vi "Tiling.vi"() -> ()   [LabVIEW 2020]
uses:
  <vilib>/DAQmx/write.llb/DAQmx Write (Analog 1D Wfm NChan NSamp).vi
  <vilib>/DAQmx/create/channels.llb/DAQmx Create Channel (AO-Voltage-Basic).vi
  <vilib>/DAQmx/configure/timing.llb/DAQmx Timing (Use Waveform).vi
  <vilib>/DAQmx/miscellaneous.llb/DAQmx Fill In Error Info.vi
  <vilib>/measure/NI_MABase.lvlib
panel:
  in  "Z step size (um) 4":dbl=0.2
  in  "Sawtooth Offset 4":dbl=0.005 format="%.2p"
  in  "Camera trigger delay (degrees) 4":dbl=-5.0 format="%.2p"
  out "# Samples written per channel 4":u32=1000
  in  "Stop Analog Signal 4":bool
  in  "Sawtooth Phase 4":dbl=180.0 format="%.2p"
  in  "Sawtooth Amplitude 4":dbl=0.24 format="%.2p"
  in  "Z step size (um) 3":dbl=0.2
  in  "Sawtooth Offset 3":dbl=0.005 format="%.2p"
  in  "Camera trigger delay (degrees) 3":dbl=-5.0 format="%.2p"
  out "# Samples written per channel 3":u32=1000
  in  "Stop Analog Signal 3":bool
  in  "Sawtooth Phase 3":dbl=180.0 format="%.2p"
  in  "Sawtooth Amplitude 3":dbl=0.24 format="%.2p"
  in  "Z step size (um) 2":dbl=0.2
  in  "Sawtooth Offset 2":dbl=0.005 format="%.2p"
  in  "Camera trigger delay (degrees) 2":dbl=-5.0 format="%.2p"
  out "# Samples written per channel 2":u32=1000
  in  "Stop Analog Signal 2":bool
  in  "Sawtooth Phase 2":dbl=180.0 format="%.2p"
  in  "Sawtooth Amplitude 2":dbl=0.24 format="%.2p"
  out "Z Position":dbl
  out "X Position":dbl=3.2928906249999996
  out "Y Position":dbl=0.7058199999999999
  out "Error out":errorcluster
  in  "Disable All Axis":bool
  in  "Sawtooth Amplitude":dbl=0.24 format="%.2p"
  in  "Sawtooth Phase":dbl=180.0 format="%.2p"
  in  "Stop Analog Signal":bool
  out "# Samples written per channel":u32=1000
  in  "Exposure time (ms)":dbl=1000.0
  in  "Camera trigger delay (degrees)":dbl=-5.0 format="%.2p"
  in  "Sawtooth Offset":dbl=0.005 format="%.2p"
  in  "Z step size (um)":dbl=0.2
  out "Number of Slices":dbl=100.0
  in  "Input will be multiplied by 5":dbl=20.0
  out "GetFirmwareVersion 2":string="3.03\r"
  out "Connected":bool=TRUE
  in  "SPIIPLUSCOM660Lib.IAsyncChannel":refnum<k7>
  # "2x2 Tiling, 1.3mm x 1.3 mm x 0.5 mm Voxel"
  # "Zstack parameters"
  # "Parameters for analog input to Voice coil"
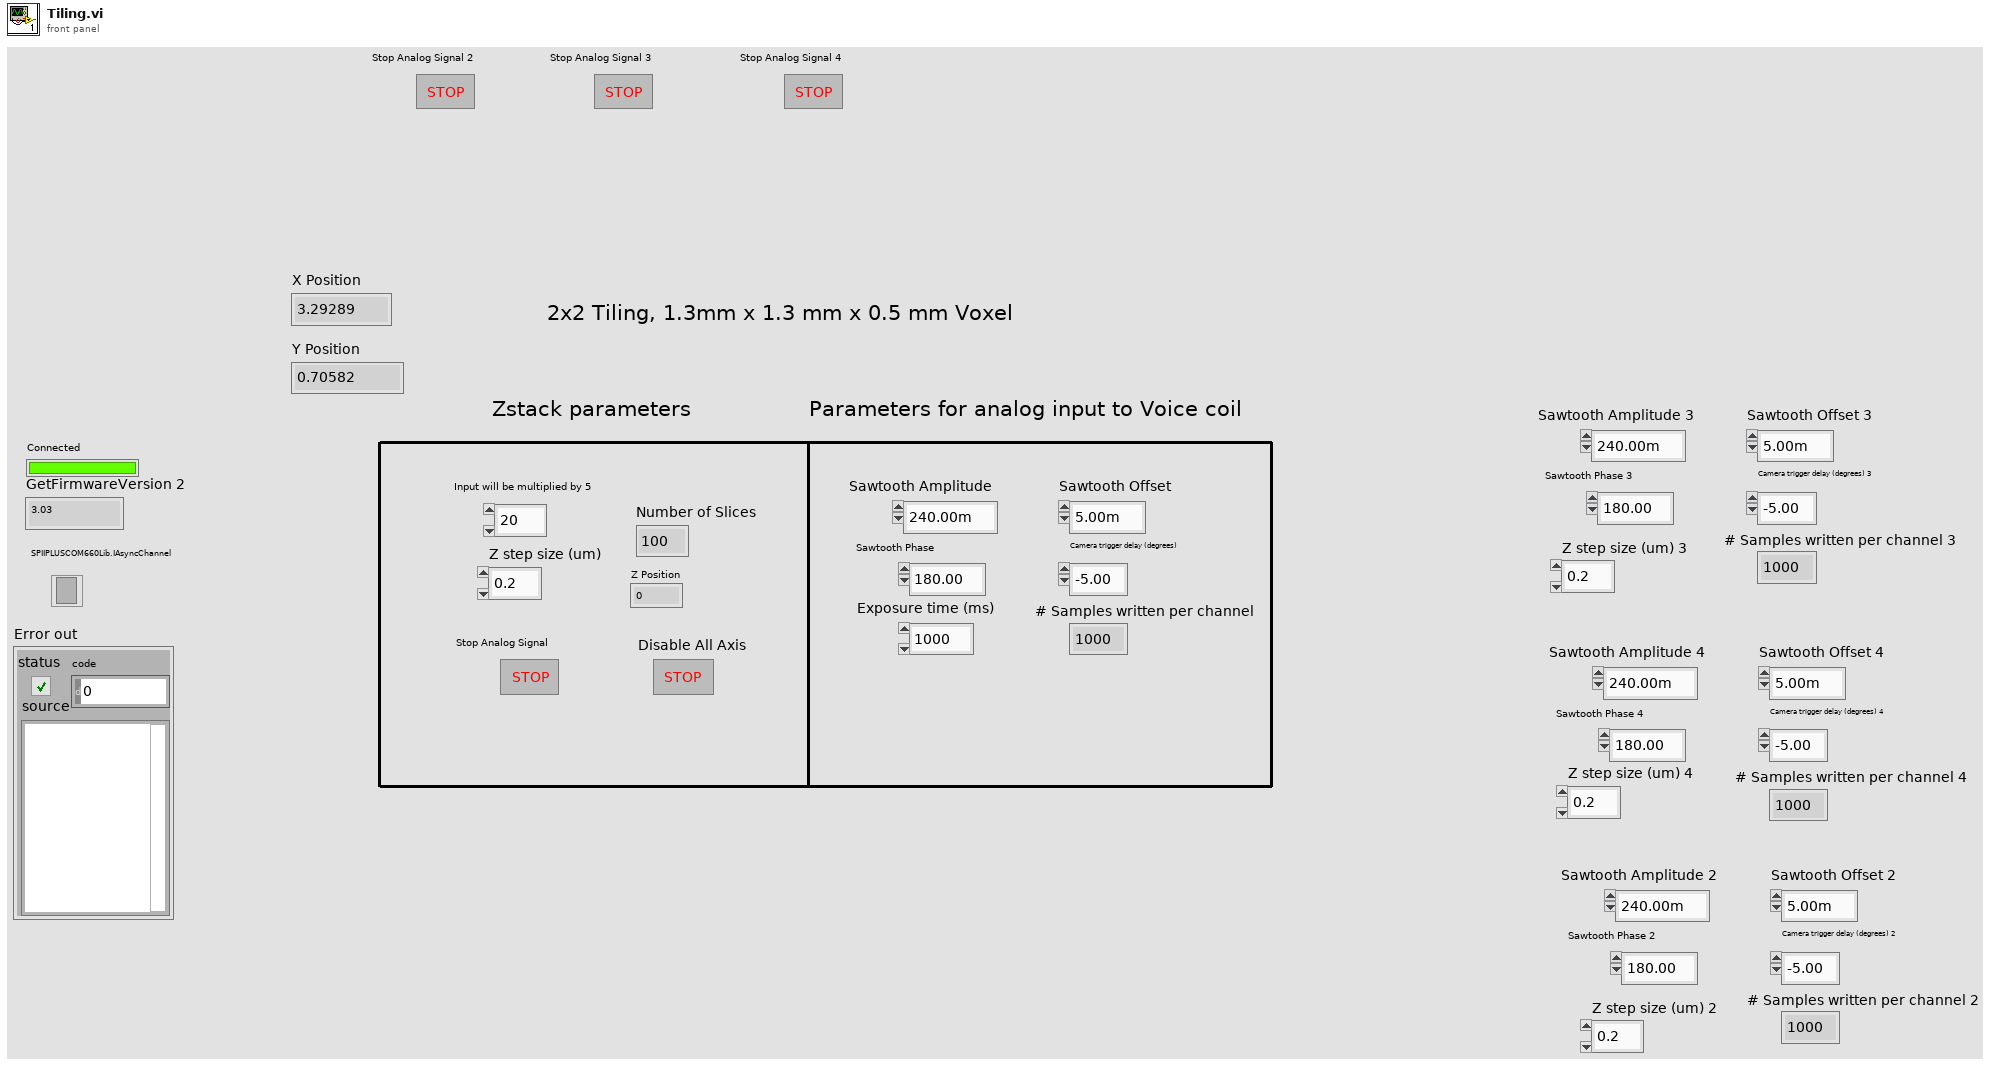
[diagram p1: front panel]
diagram:
  n1 = flat-sequence {
    tunnel: [w12] -> w9
    tunnel: [w11] -> w8
    tunnel: w9 -> [w22]
    tunnel: w8 -> [w21]
    tunnel: [w19] -> w7
    tunnel: [w18] -> w6
    tunnel: w7 -> [w29]
    tunnel: w6 -> [w30]
    tunnel: [w39] -> w5
    tunnel: [w38] -> w4
    tunnel: [w37] -> w3
    tunnel: w5 -> [w570]
    tunnel: w4 -> [w569]
    tunnel: [w568] -> w2
    tunnel: [w567] -> w1
    tunnel: w3 -> [_]
    tunnel: w2 -> [w572]
    tunnel: w1 -> [w571]
    frame #0 {
      n2 = Automation Open(Automation Refnum="SPIIPLUSCOM660Lib.IAsyncChannel") -> (Automation Refnum=w17:refnum<k7>)  [unwired: 3 in, 1 out]
      n3 = property class="IAsyncChannel"(reference=w17) -> (reference out=w16:refnum<k7>, error out=w10:errorcluster, "ACSC_SOCKET_STREAM_PORT"=w14:i32)  [unwired: 1 in]
      n4 = invoke class="IAsyncChannel" method="OpenCommEthernetTCP"(reference=w16, error in=w10, "Address"="10.0.0.100", "Port"=w14) -> (reference out=w12:refnum<k7>, error out=w11:errorcluster)  [unwired: 1 in, 3 out]
    }
    frame #1 {
      n5 = invoke class="IAsyncChannel" method="GetFirmwareVersion"(reference=w22, error in=w21, "CallType"=u64 0, "pWait"=variant) -> (reference out=w19:refnum<k7>, error out=w18:errorcluster, "GetFirmwareVersion"=w24:string)  [unwired: 1 in, 2 out]
      "GetFirmwareVersion 2" <- w24
      n6 = Empty String/Path?(string/path=w24) -> (empty?=w23:bool)
      n7 = Not(x=w23) -> (.not. x?=→"Connected":bool)
    }
    frame #2 {
      n8 = property class="IAsyncChannel"(reference=w29, error in=w30) -> (reference out=w36:refnum<k7>, error out=w35:errorcluster, "ACSC_AXIS_2"=w37:i32)
      n9 = property class="IAsyncChannel"(reference=w29, error in=w30) -> (reference out=w34:refnum<k7>, error out=w33:errorcluster, "ACSC_AXIS_0"=w32:i32)
      n10 = property class="IAsyncChannel"(reference=w29, error in=w30) -> (reference out=w28:refnum<k7>, error out=w27:errorcluster, "ACSC_AXIS_1"=w31:i32)
      n11 = while {
        shift-right: [w177] -> w39
        shift-left: w36 -> [w158]
        shift-right: [w176] -> w38
        shift-left: w35 -> [w157]
        tunnel: w37 -> [w151]
        tunnel: w32 -> [w44]
        tunnel: w31 -> [w51]
        shift-right: [w74] -> _
        shift-left: w33 -> [w163]
        shift-right: [w75] -> _
        shift-left: w34 -> [w164]
        shift-right: [w77] -> _
        shift-left: w28 -> [w79]
        shift-right: [w76] -> _
        shift-left: w27 -> [w78]
        stop <- "Disable All Axis" stop-if-true
        n12 = invoke class="IAsyncChannel" method="GetRPosition"(reference=w79, error in=w78, "Axis"=w51, "CallType"=u64 0, "pWait"=variant) -> (reference out=w57:refnum<k7>, error out=w56:errorcluster, "GetRPosition"=→"Y Position":dbl)  [unwired: 1 in, 3 out]
        n13 = invoke class="IAsyncChannel" method="GetRPosition"(reference=w164, error in=w163, "Axis"=w44, "CallType"=u64 0, "pWait"=variant) -> (reference out=w61:refnum<k7>, error out=w60:errorcluster, "GetRPosition"=→"X Position":dbl)  [unwired: 1 in, 3 out]
        n14 = invoke class="IAsyncChannel" method="GetRPosition"(reference=w158, error in=w157, "Axis"=w151, "CallType"=u64 0, "pWait"=variant) -> (reference out=w156:refnum<k7>, error out=w155:errorcluster, "GetRPosition"=→"Z Position":dbl)  [unwired: 1 in, 3 out]
        n15 = invoke class="IAsyncChannel" method="Enable"(reference=w57, error in=w56, "Axis"=w51, "CallType"=u64 0, "pWait"=variant) -> (reference out=w55:refnum<k7>, error out=w54:errorcluster)  [unwired: 1 in, 4 out]
        n16 = invoke class="IAsyncChannel" method="Enable"(reference=w61, error in=w60, "Axis"=w44, "CallType"=u64 0, "pWait"=variant) -> (reference out=w48:refnum<k7>, error out=w47:errorcluster)  [unwired: 1 in, 4 out]
        n17 = invoke class="IAsyncChannel" method="Enable"(reference=w156, error in=w155, "Axis"=w151, "CallType"=u64 0, "pWait"=variant) -> (reference out=w174:refnum<k7>, error out=w173:errorcluster)  [unwired: 1 in, 4 out]
        n18 = invoke class="IAsyncChannel" method="WaitMotorEnabled"(reference=w55, error in=w54, "Axis"=w51, "State"=1, "Timeout"=20000) -> (reference out=w53:refnum<k7>, error out=w52:errorcluster)  [unwired: 1 in, 4 out]
        n19 = invoke class="IAsyncChannel" method="WaitMotorEnabled"(reference=w48, error in=w47, "Axis"=w44, "State"=1, "Timeout"=20000) -> (reference out=w46:refnum<k7>, error out=w45:errorcluster)  [unwired: 1 in, 4 out]
        n20 = invoke class="IAsyncChannel" method="WaitMotorEnabled"(reference=w174, error in=w173, "Axis"=w151, "State"=1, "Timeout"=20000) -> (reference out=w168:refnum<k7>, error out=w167:errorcluster)  [unwired: 1 in, 4 out]
        n21 = flat-sequence {
          tunnel: w168 -> [w234]
          tunnel: w167 -> [w233]
          tunnel: w151 -> [w183]
          tunnel: w46 -> [w184]
          tunnel: w45 -> [w185]
          tunnel: w44 -> [w186]
          tunnel: w53 -> [w182]
          tunnel: w52 -> [w181]
          tunnel: w51 -> [w180]
          tunnel: [w236] -> w135
          tunnel: [w235] -> w134
          tunnel: [w186] -> w133
          tunnel: [w185] -> w130
          tunnel: [w184] -> w129
          tunnel: [w183] -> w125
          tunnel: [w182] -> w117
          tunnel: [w181] -> w116
          tunnel: [w180] -> w115
          tunnel: ["Exposure time (ms)"] -> w73
          tunnel: ["Input will be multiplied by 5"] -> w66
          tunnel: w135 -> [w283]
          tunnel: w134 -> [w282]
          tunnel: w133 -> [w269]
          tunnel: [w283] -> w132
          tunnel: [w282] -> w131
          tunnel: w130 -> [w268]
          tunnel: w129 -> [w267]
          tunnel: [w274] -> w128
          tunnel: [w273] -> w127
          tunnel: [w269] -> w126
          tunnel: w125 -> [w281]
          tunnel: [w281] -> w124
          tunnel: w117 -> [w280]
          tunnel: w116 -> [w279]
          tunnel: w115 -> [w278]
          tunnel: [w280] -> w114
          tunnel: [w279] -> w113
          tunnel: [w278] -> w112
          tunnel: w73 -> [w277]
          tunnel: [w277] -> w72
          tunnel: [w276] -> w67
          tunnel: w66 -> [w276]
          tunnel: w132 -> [w296]
          tunnel: w131 -> [w295]
          tunnel: w128 -> [w291]
          tunnel: w127 -> [w290]
          tunnel: w126 -> [w289]
          tunnel: w124 -> [w292]
          tunnel: [w294] -> w123
          tunnel: [w293] -> w122
          tunnel: [w292] -> w121
          tunnel: w114 -> [w288]
          tunnel: w113 -> [w287]
          tunnel: w112 -> [w286]
          tunnel: [w291] -> w111
          tunnel: [w290] -> w110
          tunnel: [w289] -> w109
          tunnel: [w288] -> w108
          tunnel: [w287] -> w107
          tunnel: [w286] -> w106
          tunnel: w72 -> [w285]
          tunnel: [w285] -> w71
          tunnel: w67 -> [w284]
          tunnel: [w284] -> w65
          tunnel: w123 -> [w373]
          tunnel: w122 -> [w372]
          tunnel: w121 -> [w374]
          tunnel: [w374] -> w120
          tunnel: [w373] -> w119
          tunnel: [w372] -> w118
          tunnel: w111 -> [w366]
          tunnel: w110 -> [w365]
          tunnel: w109 -> [w364]
          tunnel: w108 -> [w371]
          tunnel: w107 -> [w370]
          tunnel: w106 -> [w367]
          tunnel: [w369] -> w105
          tunnel: [w368] -> w104
          tunnel: [w367] -> w103
          tunnel: [w366] -> w102
          tunnel: [w365] -> w101
          tunnel: [w364] -> w100
          tunnel: w71 -> [w363]
          tunnel: [w363] -> w70
          tunnel: w65 -> [w362]
          tunnel: [w362] -> w64
          tunnel: w120 -> [w390]
          tunnel: w119 -> [w389]
          tunnel: w118 -> [w388]
          tunnel: w105 -> [w394]
          tunnel: w104 -> [w395]
          tunnel: w103 -> [w393]
          tunnel: w102 -> [w398]
          tunnel: w101 -> [w397]
          tunnel: w100 -> [w396]
          tunnel: [w398] -> w99
          tunnel: [w397] -> w98
          tunnel: [w396] -> w97
          tunnel: [w395] -> w96
          tunnel: [w394] -> w95
          tunnel: [w393] -> w94
          tunnel: [w392] -> w88
          tunnel: [w391] -> w87
          tunnel: [w390] -> w85
          tunnel: w70 -> [w387]
          tunnel: [w387] -> w69
          tunnel: w64 -> [w386]
          tunnel: [w386] -> w63
          tunnel: w99 -> [w476]
          tunnel: w98 -> [w475]
          tunnel: w97 -> [w469]
          tunnel: w96 -> [w474]
          tunnel: w95 -> [w473]
          tunnel: w94 -> [w472]
          tunnel: [w474] -> w93
          tunnel: [w473] -> w92
          tunnel: [w472] -> w91
          tunnel: [w471] -> w90
          tunnel: [w470] -> w89
          tunnel: w88 -> [w466]
          tunnel: w87 -> [w467]
          tunnel: [w468] -> w86
          tunnel: w85 -> [w468]
          tunnel: [w467] -> w84
          tunnel: [w466] -> w83
          tunnel: w69 -> [w465]
          tunnel: [w465] -> w68
          tunnel: w63 -> [w464]
          tunnel: [w464] -> w62
          tunnel: [w490] -> w176
          tunnel: [w491] -> w177
          tunnel: w93 -> [w494]
          tunnel: w92 -> [w493]
          tunnel: w91 -> [w492]
          tunnel: w90 -> [w496]
          tunnel: w89 -> [w495]
          tunnel: w86 -> [w499]
          tunnel: w84 -> [w497]
          tunnel: w83 -> [w498]
          tunnel: [w496] -> w75
          tunnel: [w495] -> w74
          tunnel: [w494] -> w82
          tunnel: [w493] -> w81
          tunnel: [w492] -> w80
          tunnel: w68 -> [w489]
          tunnel: w62 -> [w488]
          frame #0 {
            w203 = cluster{"Fs":dbl, "#s":dbl} {"Fs"=1000.0, "#s"=1000.0} ("sampling info")
            w226 = 10123 items=["Finite Samples"=10178, "Continuous Samples"=10123, "Hardware Timed Single Point"=12522] ("sample mode")
            n22 = property class="IAsyncChannel"(reference=w234, error in=w233) -> (reference out=w197:refnum<k7>, error out=w196:errorcluster, "ACSC_AMF_RELATIVE"=w193:i32)
            n23 = Divide(x=1000.0, y="Exposure time (ms)") -> (x/y=w202:dbl)
            n24 = invoke class="IAsyncChannel" method="MultiPoint"(reference=w197, error in=w196, "Flags"=w193, "Axis"=w183, "Dwell"="Exposure time (ms)", "CallType"=u64 0, "pWait"=variant) -> (reference out=w192:refnum<k7>, error out=w191:errorcluster)  [unwired: 1 in, 6 out]
            n25 = Multiply(x="Input will be multiplied by 5", y=5.0) -> (x*y=→"Number of Slices":dbl)
            n26 = call-poly <vilib>:"DAQmx Create Virtual Channel.vi"("physical channels"=tag "Dev1/ao0:2") -> ("task out"=w228:refnum<k21>, "error out"=w227:errorcluster)  [unwired: 13 in]
            n27 = call <vilib>:"Square Waveform.vi"("duty cycle (%)"=10.0, "offset"=2.5, "sampling info"=w203, "phase"="Camera trigger delay (degrees)", "amplitude"=2.5, "frequency"=w202) -> ("signal out"=w210:waveform(dbl))  [unwired: 4 in, 1 out]
            n28 = call <vilib>:"Square Waveform.vi"("duty cycle (%)"=93.0, "offset"=2.5, "sampling info"=w203, "phase"=-30.0, "amplitude"=2.5, "frequency"=w202) -> ("signal out"=w201:waveform(dbl))  [unwired: 4 in, 1 out]
            n29 = call <vilib>:"Sawtooth Waveform.vi"("offset"="Sawtooth Offset", "sampling info"=w203, "phase"="Sawtooth Phase", "amplitude"="Sawtooth Amplitude", "frequency"=w202) -> ("signal out"=w211:waveform(dbl))  [unwired: 5 in, 1 out]
            n30 = for {
              N: "Input will be multiplied by 5" -> [_]
              tunnel: w183 -> [w239]
              shift-right: [w241] -> w190
              shift-left: w192 -> [w243]
              shift-right: [w240] -> w189
              shift-left: w191 -> [w242]
              tunnel: "Exposure time (ms)" -> [w237]
              n31 = for {
                N: 5 -> [_]
                tunnel: w239 -> [w254]
                shift-right: [w249] -> w241
                shift-left: w243 -> [w253]
                shift-right: [w248] -> w240
                shift-left: w242 -> [w252]
                tunnel: w237 -> [w244]
                n32 = Divide(x="Z step size (um)", y=1000.0) -> (x/y=w245:dbl)
                n33 = invoke class="IAsyncChannel" method="AddPoint"(reference=w253, error in=w252, "Axis"=w254, "Point"=w245, "CallType"=u64 0, "pWait"=variant) -> (reference out=w249:refnum<k7>, error out=w248:errorcluster)  [unwired: 1 in, 5 out]
                n34 = Wait (ms)(milliseconds to wait=w244) -> ()  [unwired: 1 out]
              }
            }
            n35 = Build Array(w211, w210, w201) -> (w200:waveform(dbl)[])
            n36 = call-poly <vilib>:"DAQmx Timing.vi"("task/channels in"=w228, "sample mode"=w226, "waveform"=w211, "error in"=w227) -> ("task out"=w223:refnum<k21>, "error out"=w222:errorcluster)  [unwired: 10 in]
            n37 = call-poly <vilib>:"DAQmx Write.vi"("task/channels in"=w223, "auto start"=TRUE, "data"=w200, "timeout"=0.0, "error in"=w222) -> ("task out"=w224:refnum<k21>, "number of samples written per channel"=→"# Samples written per channel":u32, "error out"=w225:errorcluster)  [unwired: 8 in]
            n38 = while {
              shift-right: [w256] -> w219
              shift-left: w224 -> [w259]
              shift-right: [w257] -> w220
              shift-left: w225 -> [w258]
              stop <- "Stop Analog Signal" stop-if-true
              n39 = call <vilib>:"DAQmx Is Task Done.vi"("task/channels in"=w259, "error in"=w258) -> ("task out"=w256:refnum<k21>, "error out"=w257:errorcluster)  [unwired: 11 in, 1 out]
            }
            n40 = invoke class="IAsyncChannel" method="EndSequence"(reference=w190, error in=w189, "Axis"=w183, "CallType"=u64 0, "pWait"=variant) -> (reference out=w236:refnum<k7>, error out=w235:errorcluster)  [unwired: 1 in, 4 out]
            n41 = call <vilib>:"DAQmx Stop Task.vi"("task/channels in"=w219, "error in"=w220) -> ("task out"=w229:refnum<k21>, "error out"=w230:errorcluster)  [unwired: 12 in]
            n42 = call <vilib>:"DAQmx Clear Task.vi"("task in"=w229, "error in"=w230) -> ()  [unwired: 13 in, 1 out]
          }
          frame #1 {
            n43 = property class="IAsyncChannel"(reference=w267, error in=w268) -> (reference out=w266:refnum<k7>, error out=w265:errorcluster, "ACSC_AMF_RELATIVE"=w264:i32)
            n44 = invoke class="IAsyncChannel" method="MultiPoint"(reference=w266, error in=w265, "Flags"=w264, "Axis"=w269, "Dwell"=0.5 ("Point"), "CallType"=u64 0, "pWait"=variant) -> (reference out=w275:refnum<k7>, error out=w263:errorcluster)  [unwired: 1 in, 6 out]
            n45 = invoke class="IAsyncChannel" method="AddPoint"(reference=w275, error in=w263, "Axis"=w269, "Point"=0.5, "CallType"=u64 0, "pWait"=variant) -> (reference out=w274:refnum<k7>, error out=w273:errorcluster)  [unwired: 1 in, 5 out]
          }
          frame #2 {
            w311 = cluster{"Fs":dbl, "#s":dbl} {"Fs"=1000.0, "#s"=1000.0} ("sampling info")
            w334 = 10123 items=["Finite Samples"=10178, "Continuous Samples"=10123, "Hardware Timed Single Point"=12522] ("sample mode")
            n46 = property class="IAsyncChannel"(reference=w296, error in=w295) -> (reference out=w305:refnum<k7>, error out=w304:errorcluster, "ACSC_AMF_RELATIVE"=w301:i32)
            n47 = Divide(x=1000.0, y=w285) -> (x/y=w310:dbl)
            n48 = invoke class="IAsyncChannel" method="MultiPoint"(reference=w305, error in=w304, "Flags"=w301, "Axis"=w292, "Dwell"=w285, "CallType"=u64 0, "pWait"=variant) -> (reference out=w300:refnum<k7>, error out=w299:errorcluster)  [unwired: 1 in, 6 out]
            n49 = call-poly <vilib>:"DAQmx Create Virtual Channel.vi"("physical channels"=tag "Dev1/ao0:2") -> ("task out"=w336:refnum<k21>, "error out"=w335:errorcluster)  [unwired: 13 in]
            n50 = call <vilib>:"Square Waveform.vi"("duty cycle (%)"=93.0, "offset"=2.5, "sampling info"=w311, "phase"=-30.0, "amplitude"=2.5, "frequency"=w310) -> ("signal out"=w309:waveform(dbl))  [unwired: 4 in, 1 out]
            n51 = call <vilib>:"Sawtooth Waveform.vi"("offset"="Sawtooth Offset 2", "sampling info"=w311, "phase"="Sawtooth Phase 2", "amplitude"="Sawtooth Amplitude 2", "frequency"=w310) -> ("signal out"=w319:waveform(dbl))  [unwired: 5 in, 1 out]
            n52 = call <vilib>:"Square Waveform.vi"("duty cycle (%)"=10.0, "offset"=2.5, "sampling info"=w311, "phase"="Camera trigger delay (degrees) 2", "amplitude"=2.5, "frequency"=w310) -> ("signal out"=w318:waveform(dbl))  [unwired: 4 in, 1 out]
            n53 = for {
              N: w284 -> [_]
              tunnel: w292 -> [w341]
              shift-right: [w343] -> w298
              shift-left: w300 -> [w345]
              shift-right: [w342] -> w297
              shift-left: w299 -> [w344]
              tunnel: w285 -> [w339]
              n54 = for {
                N: 5 -> [_]
                tunnel: w341 -> [w356]
                shift-right: [w351] -> w343
                shift-left: w345 -> [w355]
                shift-right: [w350] -> w342
                shift-left: w344 -> [w354]
                tunnel: w339 -> [w346]
                n55 = Divide(x="Z step size (um) 2", y=1000.0) -> (x/y=w347:dbl)
                n56 = invoke class="IAsyncChannel" method="AddPoint"(reference=w355, error in=w354, "Axis"=w356, "Point"=w347, "CallType"=u64 0, "pWait"=variant) -> (reference out=w351:refnum<k7>, error out=w350:errorcluster)  [unwired: 1 in, 5 out]
                n57 = Wait (ms)(milliseconds to wait=w346) -> ()  [unwired: 1 out]
              }
            }
            n58 = Build Array(w319, w318, w309) -> (w308:waveform(dbl)[])
            n59 = call-poly <vilib>:"DAQmx Timing.vi"("task/channels in"=w336, "sample mode"=w334, "waveform"=w319, "error in"=w335) -> ("task out"=w331:refnum<k21>, "error out"=w330:errorcluster)  [unwired: 10 in]
            n60 = call-poly <vilib>:"DAQmx Write.vi"("task/channels in"=w331, "auto start"=TRUE, "data"=w308, "timeout"=0.0, "error in"=w330) -> ("task out"=w332:refnum<k21>, "number of samples written per channel"=→"# Samples written per channel 2":u32, "error out"=w333:errorcluster)  [unwired: 8 in]
            n61 = while {
              shift-right: [w358] -> w327
              shift-left: w332 -> [w361]
              shift-right: [w359] -> w328
              shift-left: w333 -> [w360]
              stop <- "Stop Analog Signal 2" stop-if-true
              n62 = call <vilib>:"DAQmx Is Task Done.vi"("task/channels in"=w361, "error in"=w360) -> ("task out"=w358:refnum<k21>, "error out"=w359:errorcluster)  [unwired: 11 in, 1 out]
            }
            n63 = invoke class="IAsyncChannel" method="EndSequence"(reference=w298, error in=w297, "Axis"=w292, "CallType"=u64 0, "pWait"=variant) -> (reference out=w294:refnum<k7>, error out=w293:errorcluster)  [unwired: 1 in, 4 out]
            n64 = call <vilib>:"DAQmx Stop Task.vi"("task/channels in"=w327, "error in"=w328) -> ()  [unwired: 12 in, 2 out]
          }
          frame #3 {
            n65 = property class="IAsyncChannel"(reference=w371, error in=w370) -> (reference out=w385:refnum<k7>, error out=w384:errorcluster, "ACSC_AMF_RELATIVE"=w381:i32)
            n66 = invoke class="IAsyncChannel" method="MultiPoint"(reference=w385, error in=w384, "Flags"=w381, "Axis"=w367, "Dwell"=200.0, "CallType"=u64 0, "pWait"=variant) -> (reference out=w380:refnum<k7>, error out=w379:errorcluster)  [unwired: 1 in, 6 out]
            n67 = invoke class="IAsyncChannel" method="AddPoint"(reference=w380, error in=w379, "Axis"=w367, "Point"=-0.65, "CallType"=u64 0, "pWait"=variant) -> (reference out=w368:refnum<k7>, error out=w369:errorcluster)  [unwired: 1 in, 5 out]
          }
          frame #4 {
            w413 = cluster{"Fs":dbl, "#s":dbl} {"Fs"=1000.0, "#s"=1000.0} ("sampling info")
            w436 = 10123 items=["Finite Samples"=10178, "Continuous Samples"=10123, "Hardware Timed Single Point"=12522] ("sample mode")
            n68 = property class="IAsyncChannel"(reference=w389, error in=w388) -> (reference out=w407:refnum<k7>, error out=w406:errorcluster, "ACSC_AMF_RELATIVE"=w403:i32)
            n69 = Divide(x=1000.0, y=w387) -> (x/y=w412:dbl)
            n70 = invoke class="IAsyncChannel" method="MultiPoint"(reference=w407, error in=w406, "Flags"=w403, "Axis"=w390, "Dwell"=w387, "CallType"=u64 0, "pWait"=variant) -> (reference out=w402:refnum<k7>, error out=w401:errorcluster)  [unwired: 1 in, 6 out]
            n71 = call-poly <vilib>:"DAQmx Create Virtual Channel.vi"("physical channels"=tag "Dev1/ao0:2") -> ("task out"=w438:refnum<k21>, "error out"=w437:errorcluster)  [unwired: 13 in]
            n72 = call <vilib>:"Square Waveform.vi"("duty cycle (%)"=93.0, "offset"=2.5, "sampling info"=w413, "phase"=-30.0, "amplitude"=2.5, "frequency"=w412) -> ("signal out"=w411:waveform(dbl))  [unwired: 4 in, 1 out]
            n73 = call <vilib>:"Sawtooth Waveform.vi"("offset"="Sawtooth Offset 3", "sampling info"=w413, "phase"="Sawtooth Phase 3", "amplitude"="Sawtooth Amplitude 3", "frequency"=w412) -> ("signal out"=w421:waveform(dbl))  [unwired: 5 in, 1 out]
            n74 = for {
              N: w386 -> [_]
              tunnel: w390 -> [w443]
              shift-right: [w445] -> w400
              shift-left: w402 -> [w447]
              shift-right: [w444] -> w399
              shift-left: w401 -> [w446]
              tunnel: w387 -> [w441]
              n75 = for {
                N: 5 -> [_]
                tunnel: w443 -> [w458]
                shift-right: [w453] -> w445
                shift-left: w447 -> [w457]
                shift-right: [w452] -> w444
                shift-left: w446 -> [w456]
                tunnel: w441 -> [w448]
                n76 = Divide(x="Z step size (um) 3", y=1000.0) -> (x/y=w449:dbl)
                n77 = invoke class="IAsyncChannel" method="AddPoint"(reference=w457, error in=w456, "Axis"=w458, "Point"=w449, "CallType"=u64 0, "pWait"=variant) -> (reference out=w453:refnum<k7>, error out=w452:errorcluster)  [unwired: 1 in, 5 out]
                n78 = Wait (ms)(milliseconds to wait=w448) -> ()  [unwired: 1 out]
              }
            }
            n79 = call <vilib>:"Square Waveform.vi"("duty cycle (%)"=10.0, "offset"=2.5, "sampling info"=w413, "phase"="Camera trigger delay (degrees) 3", "amplitude"=2.5, "frequency"=w412) -> ("signal out"=w420:waveform(dbl))  [unwired: 4 in, 1 out]
            n80 = Build Array(w421, w420, w411) -> (w410:waveform(dbl)[])
            n81 = call-poly <vilib>:"DAQmx Timing.vi"("task/channels in"=w438, "sample mode"=w436, "waveform"=w421, "error in"=w437) -> ("task out"=w433:refnum<k21>, "error out"=w432:errorcluster)  [unwired: 10 in]
            n82 = call-poly <vilib>:"DAQmx Write.vi"("task/channels in"=w433, "auto start"=TRUE, "data"=w410, "timeout"=0.0, "error in"=w432) -> ("task out"=w434:refnum<k21>, "number of samples written per channel"=→"# Samples written per channel 3":u32, "error out"=w435:errorcluster)  [unwired: 8 in]
            n83 = while {
              shift-right: [w460] -> w429
              shift-left: w434 -> [w463]
              shift-right: [w461] -> w430
              shift-left: w435 -> [w462]
              stop <- "Stop Analog Signal 3" stop-if-true
              n84 = call <vilib>:"DAQmx Is Task Done.vi"("task/channels in"=w463, "error in"=w462) -> ("task out"=w460:refnum<k21>, "error out"=w461:errorcluster)  [unwired: 11 in, 1 out]
            }
            n85 = invoke class="IAsyncChannel" method="EndSequence"(reference=w400, error in=w399, "Axis"=w390, "CallType"=u64 0, "pWait"=variant) -> (reference out=w392:refnum<k7>, error out=w391:errorcluster)  [unwired: 1 in, 4 out]
            n86 = call <vilib>:"DAQmx Stop Task.vi"("task/channels in"=w429, "error in"=w430) -> ()  [unwired: 12 in, 2 out]
          }
          frame #5 {
            n87 = property class="IAsyncChannel"(reference=w476, error in=w475) -> (reference out=w487:refnum<k7>, error out=w486:errorcluster, "ACSC_AMF_RELATIVE"=w483:i32)
            n88 = invoke class="IAsyncChannel" method="MultiPoint"(reference=w487, error in=w486, "Flags"=w483, "Axis"=w469, "Dwell"=200.0, "CallType"=u64 0, "pWait"=variant) -> (reference out=w482:refnum<k7>, error out=w481:errorcluster)  [unwired: 1 in, 6 out]
            n89 = invoke class="IAsyncChannel" method="AddPoint"(reference=w482, error in=w481, "Axis"=w469, "Point"=-0.65, "CallType"=u64 0, "pWait"=variant) -> (reference out=w471:refnum<k7>, error out=w470:errorcluster)  [unwired: 1 in, 5 out]
          }
          frame #6 {
            w514 = cluster{"Fs":dbl, "#s":dbl} {"Fs"=1000.0, "#s"=1000.0} ("sampling info")
            w537 = 10123 items=["Finite Samples"=10178, "Continuous Samples"=10123, "Hardware Timed Single Point"=12522] ("sample mode")
            n90 = property class="IAsyncChannel"(reference=w498, error in=w497) -> (reference out=w508:refnum<k7>, error out=w507:errorcluster, "ACSC_AMF_RELATIVE"=w504:i32)
            n91 = Divide(x=1000.0, y=w489) -> (x/y=w513:dbl)
            n92 = invoke class="IAsyncChannel" method="MultiPoint"(reference=w508, error in=w507, "Flags"=w504, "Axis"=w499, "Dwell"=w489, "CallType"=u64 0, "pWait"=variant) -> (reference out=w503:refnum<k7>, error out=w502:errorcluster)  [unwired: 1 in, 6 out]
            n93 = call-poly <vilib>:"DAQmx Create Virtual Channel.vi"("physical channels"=tag "Dev1/ao0:2") -> ("task out"=w539:refnum<k21>, "error out"=w538:errorcluster)  [unwired: 13 in]
            n94 = call <vilib>:"Square Waveform.vi"("duty cycle (%)"=93.0, "offset"=2.5, "sampling info"=w514, "phase"=-30.0, "amplitude"=2.5, "frequency"=w513) -> ("signal out"=w512:waveform(dbl))  [unwired: 4 in, 1 out]
            n95 = call <vilib>:"Sawtooth Waveform.vi"("offset"="Sawtooth Offset 4", "sampling info"=w514, "phase"="Sawtooth Phase 4", "amplitude"="Sawtooth Amplitude 4", "frequency"=w513) -> ("signal out"=w522:waveform(dbl))  [unwired: 5 in, 1 out]
            n96 = call <vilib>:"Square Waveform.vi"("duty cycle (%)"=10.0, "offset"=2.5, "sampling info"=w514, "phase"="Camera trigger delay (degrees) 4", "amplitude"=2.5, "frequency"=w513) -> ("signal out"=w521:waveform(dbl))  [unwired: 4 in, 1 out]
            n97 = for {
              N: w488 -> [_]
              tunnel: w499 -> [w544]
              shift-right: [w546] -> w501
              shift-left: w503 -> [w548]
              shift-right: [w545] -> w500
              shift-left: w502 -> [w547]
              tunnel: w489 -> [w542]
              n98 = for {
                N: 5 -> [_]
                tunnel: w544 -> [w559]
                shift-right: [w554] -> w546
                shift-left: w548 -> [w558]
                shift-right: [w553] -> w545
                shift-left: w547 -> [w557]
                tunnel: w542 -> [w549]
                n99 = Divide(x="Z step size (um) 4", y=1000.0) -> (x/y=w550:dbl)
                n100 = invoke class="IAsyncChannel" method="AddPoint"(reference=w558, error in=w557, "Axis"=w559, "Point"=w550, "CallType"=u64 0, "pWait"=variant) -> (reference out=w554:refnum<k7>, error out=w553:errorcluster)  [unwired: 1 in, 5 out]
                n101 = Wait (ms)(milliseconds to wait=w549) -> ()  [unwired: 1 out]
              }
            }
            n102 = Build Array(w522, w521, w512) -> (w511:waveform(dbl)[])
            n103 = call-poly <vilib>:"DAQmx Timing.vi"("task/channels in"=w539, "sample mode"=w537, "waveform"=w522, "error in"=w538) -> ("task out"=w534:refnum<k21>, "error out"=w533:errorcluster)  [unwired: 10 in]
            n104 = call-poly <vilib>:"DAQmx Write.vi"("task/channels in"=w534, "auto start"=TRUE, "data"=w511, "timeout"=0.0, "error in"=w533) -> ("task out"=w535:refnum<k21>, "number of samples written per channel"=→"# Samples written per channel 4":u32, "error out"=w536:errorcluster)  [unwired: 8 in]
            n105 = while {
              shift-right: [w561] -> w530
              shift-left: w535 -> [w564]
              shift-right: [w562] -> w531
              shift-left: w536 -> [w563]
              stop <- "Stop Analog Signal 4" stop-if-true
              n106 = call <vilib>:"DAQmx Is Task Done.vi"("task/channels in"=w564, "error in"=w563) -> ("task out"=w561:refnum<k21>, "error out"=w562:errorcluster)  [unwired: 11 in, 1 out]
            }
            n107 = invoke class="IAsyncChannel" method="EndSequence"(reference=w501, error in=w500, "Axis"=w499, "CallType"=u64 0, "pWait"=variant) -> (reference out=w491:refnum<k7>, error out=w490:errorcluster)  [unwired: 1 in, 4 out]
            n108 = call <vilib>:"DAQmx Stop Task.vi"("task/channels in"=w530, "error in"=w531) -> ()  [unwired: 12 in, 2 out]
          }
        }
        n109 = property class="IAsyncChannel"(reference=w82, error in=w81) -> (reference out=w150:refnum<k7>, error out=w149:errorcluster, "ACSC_AMF_RELATIVE"=w146:i32)
        n110 = invoke class="IAsyncChannel" method="MultiPoint"(reference=w150, error in=w149, "Flags"=w146, "Axis"=w80, "Dwell"=200.0, "CallType"=u64 0, "pWait"=variant) -> (reference out=w145:refnum<k7>, error out=w144:errorcluster)  [unwired: 1 in, 6 out]
        n111 = invoke class="IAsyncChannel" method="AddPoint"(reference=w145, error in=w144, "Axis"=w80, "Point"=0.65, "CallType"=u64 0, "pWait"=variant) -> (reference out=w140:refnum<k7>, error out=w139:errorcluster)  [unwired: 1 in, 5 out]
        n112 = invoke class="IAsyncChannel" method="Break"(reference=w140, error in=w139, "Axis"=w80, "CallType"=u64 0, "pWait"=variant) -> (reference out=w77:refnum<k7>, error out=w76:errorcluster)  [unwired: 1 in, 4 out]
      }
    }
    frame #3 {
      n113 = invoke class="IAsyncChannel" method="DisableAll"(reference=w570, error in=w569, "CallType"=u64 0, "pWait"=variant) -> (reference out=w568:refnum<k7>, error out=w567:errorcluster)  [unwired: 1 in, 3 out]
    }
    frame #4 {
      n114 = invoke class="IAsyncChannel" method="CloseComm"(reference=w572, error in=w571) -> (error out=→"Error out":errorcluster)  [unwired: 1 in, 2 out]
    }
    frame #5 {
      n115 = local write "Connected"(FALSE ("Connected")) -> ()
    }
  }
